vi "rename channel test.vi"() -> ()   [LabVIEW 2013, in "scan engine tests.lvlib"]
uses:
  scan engine tests.lvlib
  configuration/Scan Engine configuration.lvclass
  <vilib>/NI/Tag Bus/tag/tag descriptor.lvclass/tag descriptor.ctl
  <vilib>/NI/Tag Bus Module Framework/root configuration/TBM configuration.lvclass
  <vilib>/NI/Tag Bus/tag/tag descriptor.lvclass
panel:
  out "rename success":bool
  out "no err":errorcluster
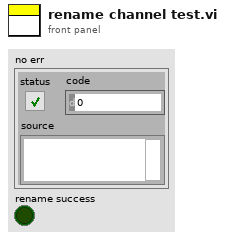
[diagram p1: front panel]
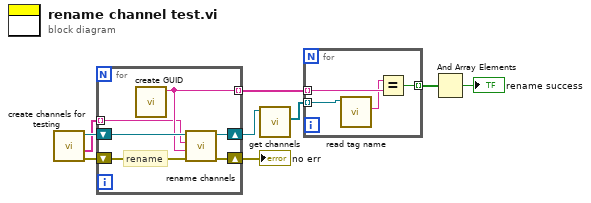
[diagram p0: block diagram]
diagram:
  n1 = call "create channels for testing.vi"() -> ("error out"=w1:errorcluster, "names"=w2:string[], "Scan Engine configuration out"=w3:refnum<class "Scan Engine configuration.lvclass">)  [unwired: 7 in, 2 out]
  n2 = for {
    shift-right: [w14] -> w4
    shift-left: w3 -> [w15]
    shift-right: [w10] -> w8
    shift-left: w1 -> [w11]
    tunnel: [w13] -> w9 mode=indexing
    tunnel: w2 -> [w12] mode=indexing
    # "rename"
    n3 = call <vilib>:"create GUID.vi"() -> ("uuid"=w13:string)  [unwired: 11 in]
    n4 = call "rename channels.vi"("error in"=w11, "new name"=w13, "old name"=w12, "Scan Engine configuration in"=w15) -> ("error out"=w10:errorcluster, "Scan Engine configuration out"=w14:refnum<class "Scan Engine configuration.lvclass">)  [unwired: 6 in]
  }
  "no err" <- w8
  n5 = call-dynamic "get channels.vi"("module configuration in"=w4) -> ("channels"=w7:refnum<class "TBM channel.lvclass">[])  [unwired: 9 in, 1 out]
  n6 = for {
    tunnel: w9 -> [w18] mode=indexing
    tunnel: w7 -> [w19] mode=indexing
    tunnel: [w16] -> w6 mode=indexing
    n7 = call <vilib>:"read tag name.vi"("system tag in"=w19) -> ("name"=w17:string)  [unwired: 8 in, 2 out]
    n8 = Equal?(x=w17, y=w18) -> (x = y?=w16:bool)
  }
  n9 = And Array Elements(Boolean array=w6) -> (logical AND=→"rename success":bool)
